vi "FPGA Reference - Close.vi"(8 "error in":errorcluster) -> (0 "error out":errorcluster)   [LabVIEW 2024, in "FPGA Interface.lvlib"]
uses:
  FPGA Interface.lvlib
  FPGA Ref Action.ctl
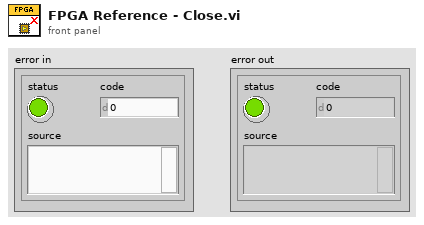
[diagram p1: front panel]
types:
  T1 = typedef "FPGA Interface.lvlib/FPGA Ref Action.ctl" = enum16{"Open Ref", "Get Ref", "Close Ref"}
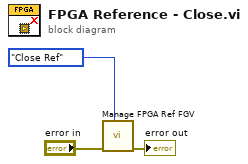
[diagram p0: block diagram]
diagram:
  n1 = call "Manage FPGA Ref FGV.vi"("FPGA Action"=FPGA_Ref_Action."Close Ref", "error in"="error in") -> ("error out"=→"error out":errorcluster)  [unwired: 8 in, 1 out]
